vi "Clear Bookmarks View.vi"(8 "Error In":errorcluster, 11 "State In":T1) -> (0 "Error Out":errorcluster, 3 "State Out":T1)   [LabVIEW 2018, in "Bookmark Manager.lvlib"]
uses:
  Bookmark Manager.lvlib
  Controls/State.ctl
  <vilib>/addons/analyzer/_analyzerctrls.llb/VIAnCtl Analysis App Info.ctl
  Controls/Bookmark.ctl
  Controls/VI Identifier.ctl
  Controls/Bookmarks Groups.ctl
  User Visible Strings.vi
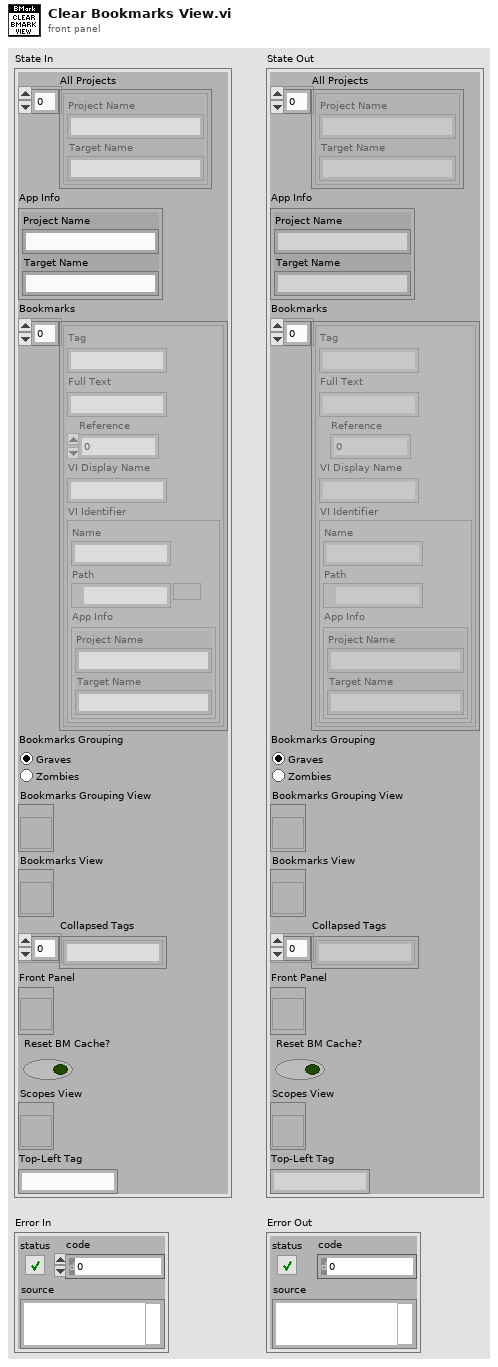
[diagram p1: front panel]
types:
  T1 = typedef "Bookmark Manager.lvlib/State.ctl" = cluster{"All Projects":T2[], "App Info":T2, "Bookmarks":T3[], "Bookmarks Grouping":T5, "Bookmarks Grouping View":refnum<vi>, "Bookmarks View":refnum<vi>, "Collapsed Tags":string[], "Front Panel":refnum<vi>, "Reset BM Cache?":bool, "Scopes View":refnum<vi>, "Top-Left Tag":string}
  T2 = typedef "VIAnCtl Analysis App Info.ctl" = cluster{"Project Name":string, "Target Name":string}
  T3 = typedef "Bookmark Manager.lvlib/Bookmark.ctl" = cluster{"Tag":string, "Full Text":string, "Reference":i32, "VI Display Name":string, "VI Identifier":T4}
  T4 = typedef "Bookmark Manager.lvlib/VI Identifier.ctl" = cluster{"Name":string, "Path":path, "App Info":T2}
  T5 = typedef "Bookmark Manager.lvlib/Bookmarks Groups.ctl" = enum32{"Graves", "Zombies"}
  T6 = enum8{"Enabled", "Disabled", "Disabled and Grayed Out"}
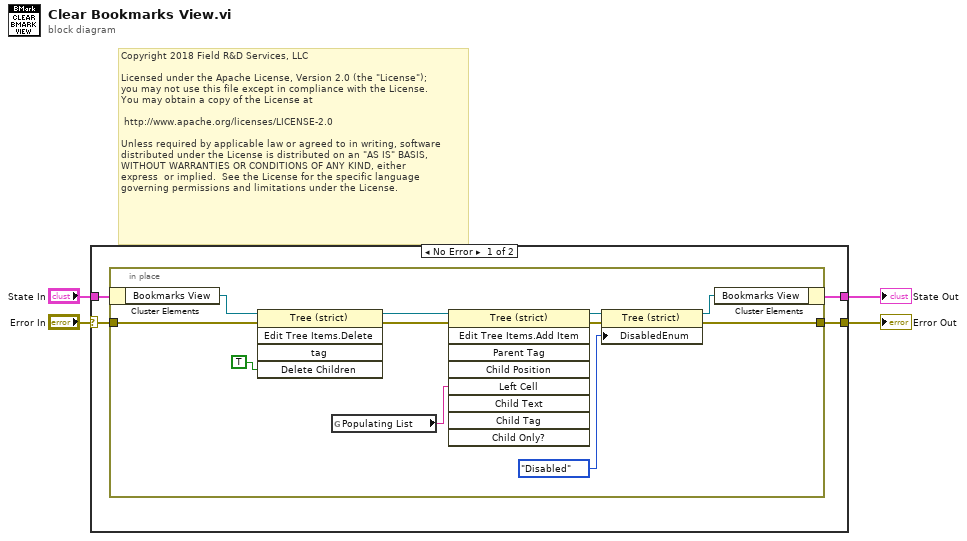
[diagram p0: block diagram]
diagram:
  # "Copyright 2018 Field R&D Services, LLC\n\nLicensed under the Apache License, Version 2.0 (the \"License\");\nyou may not use this file except in compliance with the License.\nYou may obtain a copy of the License at\n\n\thttp://www.apache.org/licenses/LICENSE-2.0\n\nUnless required by applicable law or agreed to in writing, software\ndistributed under the License is distributed on an \"AS IS\" BASIS,\nWITHOUT WARRANTIES OR CONDITIONS OF ANY KIND, either \nexpress  or implied.  See the License for the specific language \ngoverning permissions and limitations under the License."
  n1 = case shown="No Error" "Error In" {
    selector: "Error In" -> [w5 w20]
    tunnel: [w8 w20] -> w4
    tunnel: [w7 w21] -> w3
    tunnel: "State In" -> [w6 w21]
    frame No Error {
      n2 = in-place {
        in-place-border: w5 -> [w18]
        in-place-border: [w9] -> w8
        n3 = in-place-cluster #1(w6) -> ("Bookmarks View"=w19:refnum<vi>)
        n4 = invoke class="Tree (strict)" method="Edit Tree Items.Delete"(reference=w19, error in=w18, "Delete Children"=TRUE ("Delete Children?")) -> (reference out=w16:refnum<vi>, error out=w15:errorcluster)  [unwired: 2 in, 3 out]
        n5 = global read "User Visible Strings.vi" "Populating List"() -> (w14:string)
        n6 = invoke class="Tree (strict)" method="Edit Tree Items.Add Item"(reference=w16, error in=w15, "Left Cell"=w14) -> (reference out=w13:refnum<vi>, error out=w12:errorcluster)  [unwired: 6 in, 7 out]
        n7 = property class="Tree (strict)"(reference=w13, error in=w12, "DisabledEnum"=T6."Disabled" ("Disabled")) -> (reference out=w10:refnum<vi>, error out=w9:errorcluster)
        n8 = in-place-cluster #1("Bookmarks View"=w10) -> (w7:T1)
      }
    }
    frame Error {
    }
  }
  "Error Out" <- w4
  "State Out" <- w3
